vi "U8 from Pointer.vi"(4 "Type":u8, 5 "error in (no error)":errorcluster, 8 "Pointer":i32) -> (0 "error out":errorcluster, 2 "data":u8, 3 "Duplicate Pointer":i32)   [LabVIEW 2011]
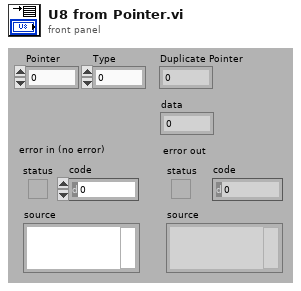
[diagram p1: front panel]
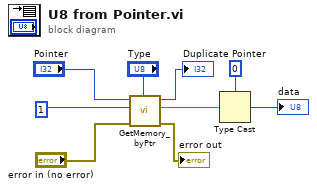
[diagram p0: block diagram]
diagram:
  n1 = call "GetMemory_byPtr.vi"("Data Type"="Type", "error in (no error)"="error in (no error)", "Data Size(1)"=1, "Pointer"="Pointer") -> ("error out"=→"error out":errorcluster, "data"=w3:string, "Duplicate Pointer"=→"Duplicate Pointer":i32)  [unwired: 2 out]
  n2 = Type Cast(type=u8 0, x=w3) -> (*(type *) &x=→"data":u8)
